vi "Keithley 6517 Read Temp and Humidity.vi"(8 "error in":T1, 11 "GPIB address":string="27") -> (0 "error out":T1, 1 "Humidity":dbl, 3 "Temp":dbl, 4 "Humidity (Text)":string, 5 "Temp (Text)":string)   [LabVIEW 2013]
doc: "This VI is used to secondary display of the Keithley 6517 and parse out the temp and humidity readings. MUST run Temp & Humidity setup VI ONCE before running this VI."
panel:
  out "secondary display":string
  # "F"
  # "%"
  # "F"
  # "%"
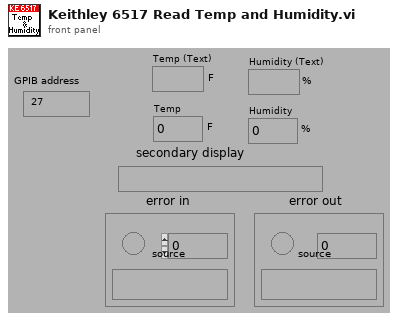
[diagram p1: front panel]
types:
  T1 = cluster{"error":bool, "code":i32, "source":string}
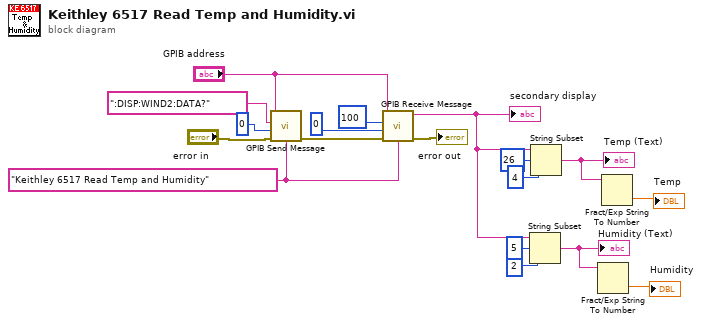
[diagram p0: block diagram]
diagram:
  w11 = "Keithley 6517 Read Temp and Humidity"
  n1 = call "GPIB Send Message.vi"("address string"="GPIB address", "write buffer"=":DISP:WIND2:DATA?", "source"=w11, "write mode (set END:0)"=0, "error in"="error in") -> ("error out"=w15:T1)  [unwired: 2 in, 2 out]
  n2 = call "GPIB Receive Message.vi"("address string"="GPIB address", "byte count"=100, "source"=w11, "read mode"=0, "error in"=w15) -> ("read buffer"=w5:string, "error out"=→"error out":T1)  [unwired: 2 in, 1 out]
  "secondary display" <- w5
  n3 = String Subset(string=w5, offset (0)=5, length (rest)=2 ("length (rest)")) -> (substring=w1:string)
  "Humidity (Text)" <- w1
  n4 = String Subset(string=w5, offset (0)=26, length (rest)=4 ("length (rest)")) -> (substring=w4:string)
  "Temp (Text)" <- w4
  n5 = Fract/Exp String To Number(string=w1) -> (number=→"Humidity":dbl)  [unwired: 3 in, 1 out]
  n6 = Fract/Exp String To Number(string=w4) -> (number=→"Temp":dbl)  [unwired: 3 in, 1 out]
